vi "1D_LDA_Time_scale_estimate.vi"(1 "Average Frequency Hz":dbl, 2 "Time":dbl[](array[numeric]), 4 "Velocity":dbl[](array[numeric])) -> (0 "Time scale estimate (s)":dbl)   [LabVIEW 2011]
uses:
  Globals/Meas_global.vi
  <vilib>/Analysis/NI_AALPro.lvlib
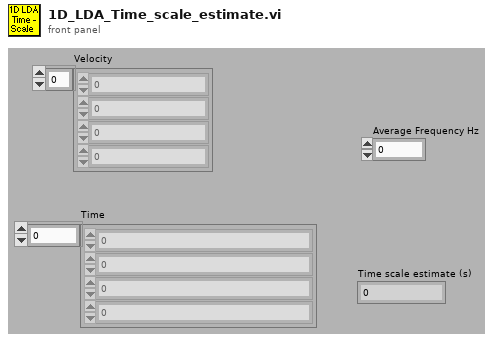
[diagram p1: front panel]
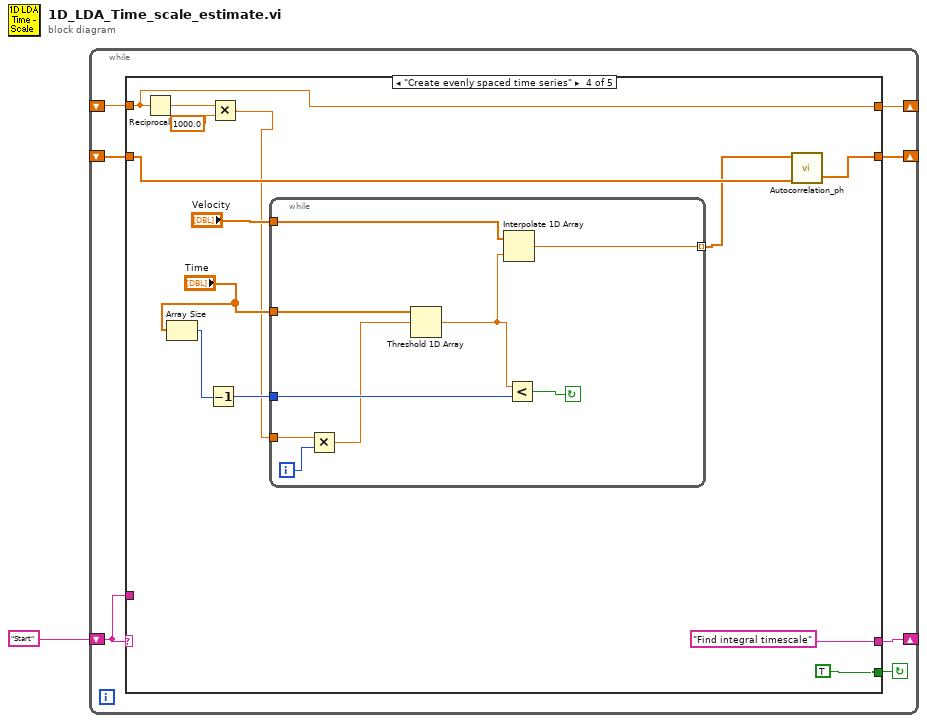
[diagram p0: block diagram]
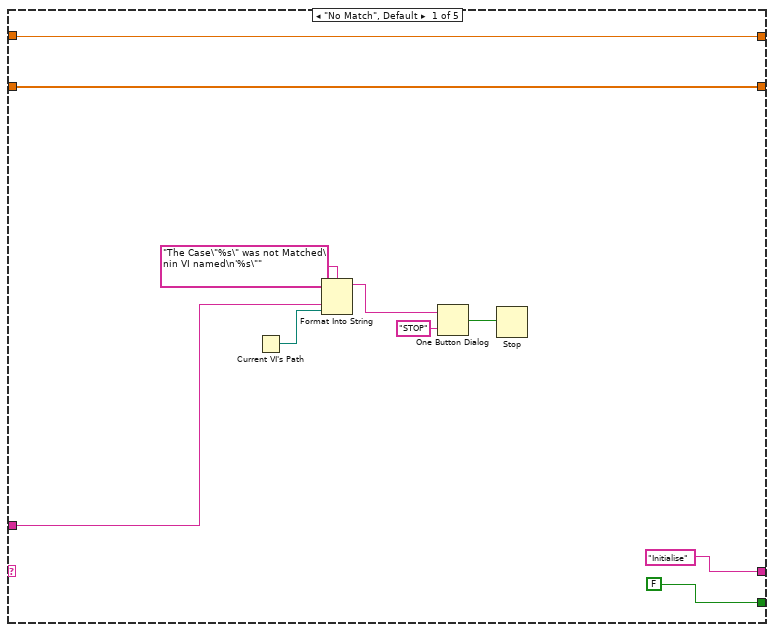
[diagram p2: hidden frame]
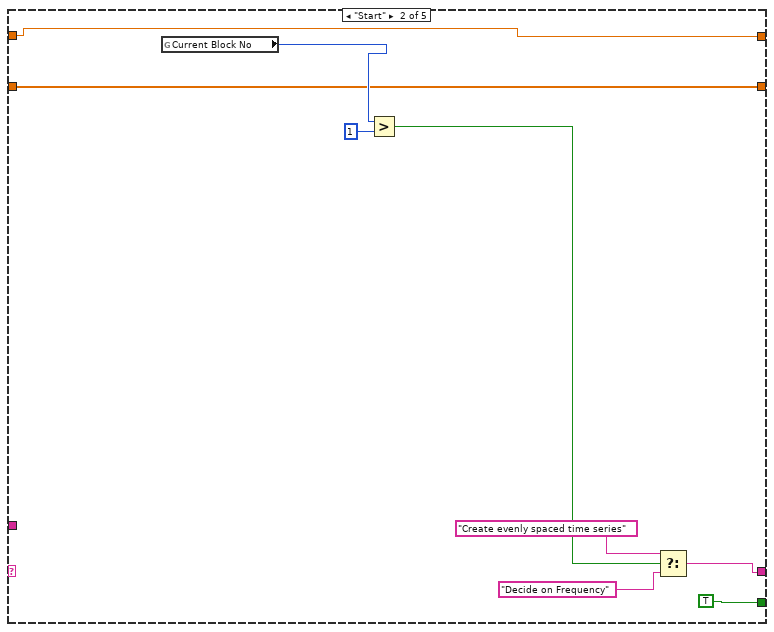
[diagram p3: hidden frame]
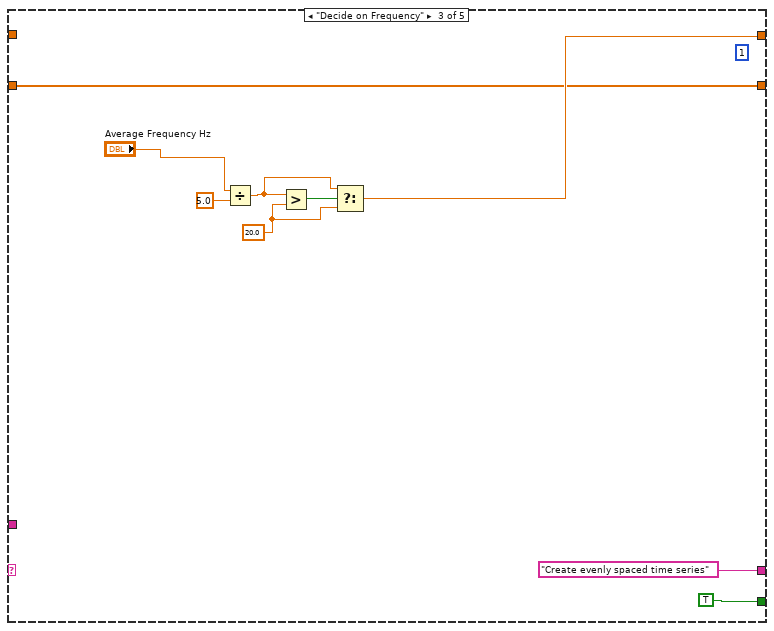
[diagram p4: hidden frame]
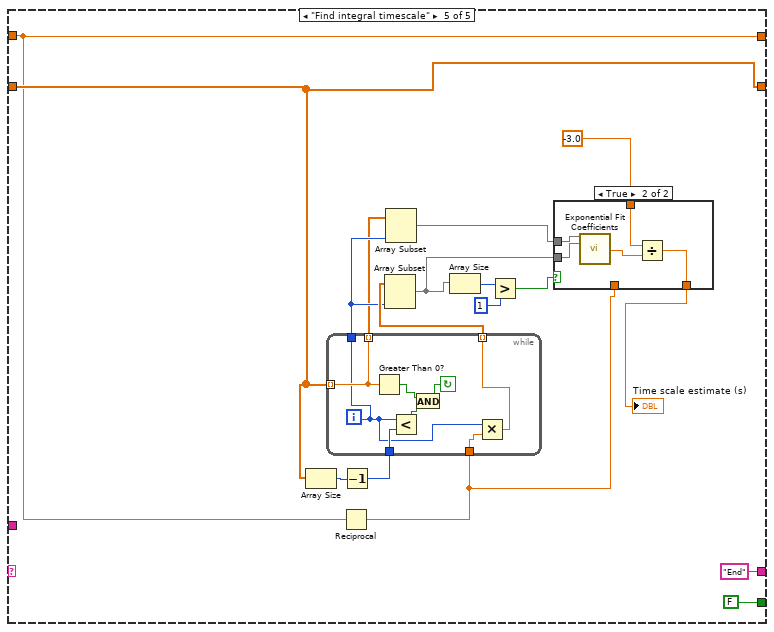
[diagram p5: hidden frame]
diagram:
  n1 = while {
    shift-left: "Start" -> [w6]
    shift-right: [w7] -> _
    shift-right: [w5] -> _
    shift-left: _ -> [w4]
    shift-right: [w3] -> _
    shift-left: _ -> [w2]
    stop <- w8 continue-if-true
    n2 = case shown="\"Create evenly spaced time series\"" w6 {
      tunnel: [FALSE TRUE TRUE TRUE FALSE] -> w8
      tunnel: ["Initialise" w26 "Create evenly spaced time series" "Find integral timescale" "End"] -> w7
      tunnel: w6 -> [w13 _ _ _ _]
      tunnel: [w10 w22 w29 w41 w67] -> w5
      tunnel: w4 -> [w10 w22 _ w41 w67]
      tunnel: [w9 w21 w28 w39 w68] -> w3
      tunnel: w2 -> [w9 w21 w28 w40 w68]
      frame "No Match", Default {
        n3 = Current VI's Path() -> (path=w12:path)
        n4 = Format Into String(format string="The Case\"%s\" was not Matched\nin VI named\n'%s\"" ("Format String"), w13, w12) -> (resulting string=w16:string)  [unwired: 2 in, 1 out]
        n5 = One Button Dialog(message=w16, button name ("OK")="STOP") -> (true=w14:bool)
        n6 = Stop(stop? (T)=w14) -> ()
      }
      frame "Start" {
        n7 = global read "Meas_global.vi" "Current Block No"() -> (w23:i32)
        n8 = Greater?(x=w23, y=1) -> (0:w25:bool)
        n9 = Select(t="Create evenly spaced time series", s=w25, f="Decide on Frequency") -> (s? t:f=w26:string)
      }
      frame "Decide on Frequency" {
        (unwired) 1 ("Current Block No")
        w31 = 20.0 ("y")
        n10 = Divide(x="Average Frequency Hz", y=5.0) -> (x/y=w32:dbl)
        n11 = Greater?(x=w32, y=w31) -> (0:w33:bool)
        n12 = Select(t=w32, s=w33, f=w31) -> (s? t:f=w29:dbl)
      }
      frame "Create evenly spaced time series" {
        n13 = Reciprocal(x=w41) -> (1/x=w43:dbl)
        n14 = Array Size(array="Time") -> (size(s)=w44:i32)
        n15 = Decrement(x=w44) -> (x-1=w45:i32)
        n16 = Multiply(x=w43, y=1000.0) -> (x*y=w37:dbl)
        n17 = while {
          tunnel: w37 -> [w57]
          tunnel: "Time" -> [w56]
          tunnel: w45 -> [w55]
          tunnel: "Velocity" -> [w53]
          tunnel: [w51] -> w38 mode=indexing
          i -> [w58]
          stop <- w54 continue-if-true
          n18 = Multiply(x=w57, y=w58) -> (x*y=w50:dbl)
          n19 = Threshold 1D Array(2:w50, 3:w56) -> (0:w52:dbl)  [unwired: 1 out]
          n20 = Interpolate 1D Array(1:w52, 2:w53) -> (0:w51:dbl)
          n21 = Less?(x=w52, y=w55) -> (x < y?=w54:bool)
        }
        n22 = call "Autocorrelation_ph.vi"("X"=w38, "Autocorrelation of X"=w40) -> ("Autocorrelation of X"=w39:dbl[])  [unwired: 3 in, 1 out]
      }
      frame "Find integral timescale" {
        n23 = Array Size(array=w68) -> (size(s)=w71:i32)
        n24 = Reciprocal(x=w67) -> (1/x=w60:dbl)
        n25 = Decrement(x=w71) -> (x-1=w72:i32)
        n26 = while {
          tunnel: w68 -> [w83] mode=indexing
          tunnel: w72 -> [w89]
          tunnel: w60 -> [w85]
          tunnel: [w84] -> w75 mode=indexing
          tunnel: [w83] -> w73 mode=indexing
          tunnel: [w82] -> w74
          i -> [w82]
          stop <- w86 continue-if-true
          n27 = Greater Than 0?(x=w83) -> (x > 0?=w88:bool)
          n28 = Less?(x=w82, y=w89) -> (x < y?=w87:bool)
          n29 = And(x=w88, y=w87) -> (x .and. y?=w86:bool)
          n30 = Multiply(x=w82, y=w85) -> (x*y=w84:dbl)
        }
        n31 = Array Subset(array=w75, length=w74) -> (w63:dbl[])  [unwired: 1 in]
        n32 = Array Subset(array=w73, length=w74) -> (w62:dbl[])  [unwired: 1 in]
        n33 = Array Size(array=w63) -> (size(s)=w66:i32)
        n34 = Greater?(x=w66, y=1) -> (0:w64:bool)
        n35 = case shown="True" w64 {
          tunnel: [w76 w80] -> w59
          tunnel: w62 -> [_ w79]
          tunnel: -3.0 ("x") -> [_ w78]
          tunnel: w63 -> [_ w77]
          tunnel: w60 -> [w76 _]
          frame False {
          }
          frame True {
            n36 = call <vilib>:"Exponential Fit Coefficients.vi"("Y"=w79, "X"=w77) -> ("damping"=w81:dbl)  [unwired: 4 in, 9 out]
            n37 = Divide(x=w78, y=w81) -> (x/y=w80:dbl)
          }
        }
        "Time scale estimate (s)" <- w59
      }
    }
  }
